vi "ma_basicErrorCode2ErrorCluster.vi"(1 "error in (no error)":errorcluster, 2 "subVI name":string, 3 "Error Code":i32) -> (0 "error out":errorcluster)   [LabVIEW 2022 SP3, in "NI_MABase.lvlib"]
uses:
  NI_MABase.lvlib
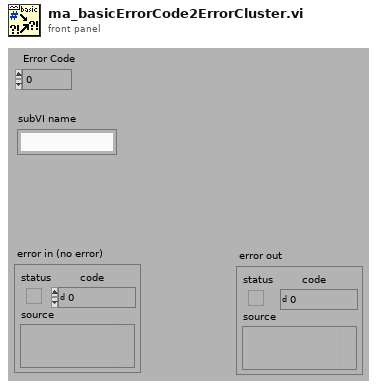
[diagram p1: front panel]
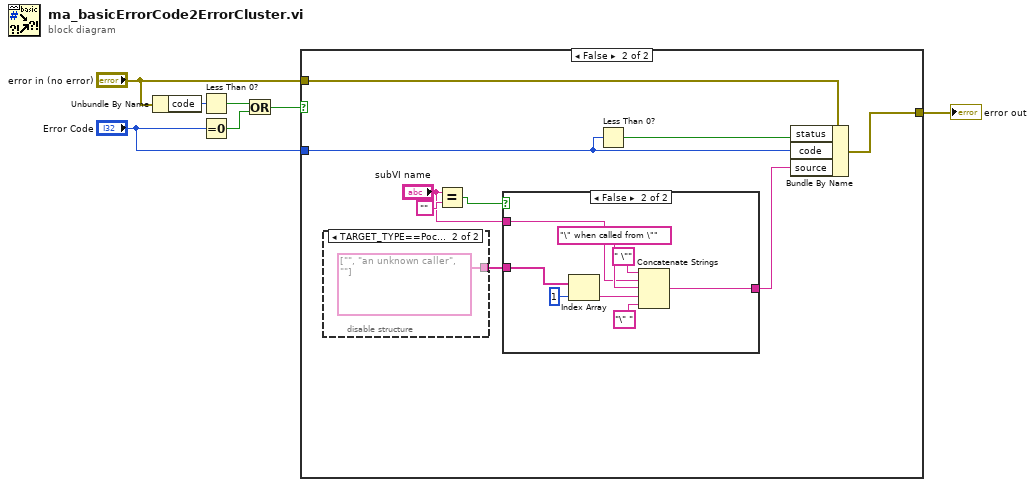
[diagram p0: block diagram]
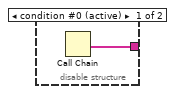
[diagram p3: hidden frame]
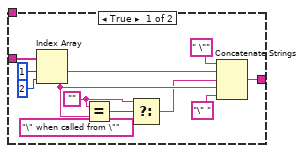
[diagram p4: hidden frame]
diagram:
  n1 = Unbundle By Name("error in (no error)") -> ("code"=w4:i32)
  n2 = Less Than 0?(x=w4) -> (x < 0?=w2:bool)
  n3 = Equal To 0?(x="Error Code") -> (x = 0?=w1:bool)
  n4 = Or(x=w2, y=w1) -> (x .or. y?=w3:bool)
  n5 = case shown="False" w3 {
    tunnel: "Error Code" -> [_ w14]
    tunnel: "error in (no error)" -> [w8 w17]
    tunnel: [w8 w16] -> w7
    frame True {
    }
    frame False {
      n6 = disable-structure shown="TARGET_TYPE==PocketPC||TARGET_TYPE==Embedded" {
        disable-tunnel: [w18 string[] ["", "an unknown caller", ""] ("call chain")] -> w9
        frame condition #0 (active) {
          n7 = Call Chain() -> (call chain=w18:string[])
        }
        frame condition #1 {
        }
      }
      n8 = Equal?(x="subVI name", y="") -> (x = y?=w10:bool)
      n9 = case shown="False" w10 {
        tunnel: [w26 w35] -> w15
        tunnel: w9 -> [w25 w34]
        tunnel: "subVI name" -> [_ w32]
        frame True {
          w22 = ""
          n10 = Index Array(array=w25, index #1=1 ("Index"), index #2=2 ("Index")) -> (element #1=w29:string, element #2=w23:string)
          n11 = Equal?(x=w22, y=w23) -> (x = y?=w24:bool)
          n12 = Select(t=w22, s=w24, f="\" when called from \"") -> (s? t:f=w20:string)
          n13 = Concatenate Strings(" \"" ("Substring"), w29, w20, w23, "\" ") -> (w26:string)
        }
        frame False {
          n14 = Index Array(array=w34, index=1 ("Index")) -> (element=w33:string)
          n15 = Concatenate Strings(" \"" ("Substring"), w32, "\" when called from \"", w33, "\" ") -> (w35:string)
        }
      }
      n16 = Less Than 0?(x=w14) -> (x < 0?=w13:bool)
      n17 = Bundle By Name(cluster=w17, "status"=w13, "code"=w14, "source"=w15) -> (w16:errorcluster)
    }
  }
  "error out" <- w7
